vi "大富翁.vi"() -> ()   [LabVIEW 2014] (continued)
                                n1451 = property on="P2 棋子" class="Bool (strict)"("Left"=1540 ("Position:Left"), "Top"=112 ("Position:Top")) -> ()  [unwired: 2 in, 2 out]
                              }
                              frame 3 {
                                n1452 = local write "剩幾天 3"(2.0 ("剩幾天 3")) -> ()
                                n1453 = local write "位置 3"(13.0 ("位置 3")) -> ()
                                n1454 = property on="入獄 3" class="Bool (strict)"("Visible"=TRUE) -> ()  [unwired: 2 in, 2 out]
                                n1455 = property on="P3 棋子" class="Bool (strict)"("Left"=1503 ("Position:Left"), "Top"=144 ("Position:Top")) -> ()  [unwired: 2 in, 2 out]
                              }
                              frame 4 {
                                n1456 = local write "剩幾天 4"(2.0 ("剩幾天 4")) -> ()
                                n1457 = local write "位置 4"(13.0 ("位置 4")) -> ()
                                n1458 = property on="入獄 4" class="Bool (strict)"("Visible"=TRUE) -> ()  [unwired: 2 in, 2 out]
                                n1459 = property on="P4 棋子" class="Bool (strict)"("Left"=1540 ("Position:Left"), "Top"=144 ("Position:Top")) -> ()  [unwired: 2 in, 2 out]
                              }
                            }
                            n1460 = call "32入獄.vi"() -> ()  [unwired: 4 in]
                          }
                        }
                      }
                      frame True {
                        # "2~5"
                        n1461 = local read "換誰?"() -> (w868:dbl)
                        n1462 = case shown="1" w868 {
                          frame 0, Default {
                          }
                          frame 1 {
                            n1463 = local write "剩幾天 1"(3.0 ("剩幾天 1")) -> ()
                            n1464 = local write "位置 1"(13.0 ("位置 1")) -> ()
                            n1465 = property on="入獄 1" class="Bool (strict)"("Visible"=TRUE) -> ()  [unwired: 2 in, 2 out]
                            n1466 = property on="P1 棋子" class="Bool (strict)"("Left"=1503 ("Position:Left"), "Top"=112 ("Position:Top")) -> ()  [unwired: 2 in, 2 out]
                          }
                          frame 2 {
                            n1467 = local write "位置 2"(13.0 ("位置 2")) -> ()
                            n1468 = local write "剩幾天 2"(3.0 ("剩幾天 2")) -> ()
                            n1469 = property on="入獄 2" class="Bool (strict)"("Visible"=TRUE) -> ()  [unwired: 2 in, 2 out]
                            n1470 = property on="P2 棋子" class="Bool (strict)"("Left"=1540 ("Position:Left"), "Top"=112 ("Position:Top")) -> ()  [unwired: 2 in, 2 out]
                          }
                          frame 3 {
                            n1471 = local write "剩幾天 3"(3.0 ("剩幾天 3")) -> ()
                            n1472 = local write "位置 3"(13.0 ("位置 3")) -> ()
                            n1473 = property on="入獄 3" class="Bool (strict)"("Visible"=TRUE) -> ()  [unwired: 2 in, 2 out]
                            n1474 = property on="P3 棋子" class="Bool (strict)"("Left"=1503 ("Position:Left"), "Top"=144 ("Position:Top")) -> ()  [unwired: 2 in, 2 out]
                          }
                          frame 4 {
                            n1475 = local write "剩幾天 4"(3.0 ("剩幾天 4")) -> ()
                            n1476 = local write "位置 4"(13.0 ("位置 4")) -> ()
                            n1477 = property on="入獄 4" class="Bool (strict)"("Visible"=TRUE) -> ()  [unwired: 2 in, 2 out]
                            n1478 = property on="P4 棋子" class="Bool (strict)"("Left"=1540 ("Position:Left"), "Top"=144 ("Position:Top")) -> ()  [unwired: 2 in, 2 out]
                          }
                        }
                        n1479 = call "入獄3天.vi"() -> ()  [unwired: 4 in]
                      }
                    }
                  }
                  frame True {
                    # "0~2%"
                    n1480 = stacked-sequence {
                      tunnel: [_ w922] -> w889
                      frame #0 {
                        n1481 = local read "換誰?"() -> (w890:dbl)
                        n1482 = case shown="4" w890 {
                          frame 0, Default {
                          }
                          frame 1 {
                            n1483 = local write "剩幾天 1"(5.0 ("剩幾天 1")) -> ()
                            n1484 = local write "位置 1"(13.0 ("位置 1")) -> ()
                            n1485 = property on="入獄 1" class="Bool (strict)"("Visible"=TRUE) -> ()  [unwired: 2 in, 2 out]
                            n1486 = property on="P1 棋子" class="Bool (strict)"("Left"=1503 ("Position:Left"), "Top"=112 ("Position:Top")) -> ()  [unwired: 2 in, 2 out]
                          }
                          frame 2 {
                            n1487 = local write "位置 2"(13.0 ("位置 2")) -> ()
                            n1488 = local write "剩幾天 2"(5.0 ("剩幾天 2")) -> ()
                            n1489 = property on="入獄 2" class="Bool (strict)"("Visible"=TRUE) -> ()  [unwired: 2 in, 2 out]
                            n1490 = property on="P2 棋子" class="Bool (strict)"("Left"=1540 ("Position:Left"), "Top"=112 ("Position:Top")) -> ()  [unwired: 2 in, 2 out]
                          }
                          frame 3 {
                            n1491 = local write "剩幾天 3"(5.0 ("剩幾天 3")) -> ()
                            n1492 = local write "位置 3"(13.0 ("位置 3")) -> ()
                            n1493 = property on="入獄 3" class="Bool (strict)"("Visible"=TRUE) -> ()  [unwired: 2 in, 2 out]
                            n1494 = property on="P3 棋子" class="Bool (strict)"("Left"=1503 ("Position:Left"), "Top"=144 ("Position:Top")) -> ()  [unwired: 2 in, 2 out]
                          }
                          frame 4 {
                            n1495 = local write "剩幾天 4"(5.0 ("剩幾天 4")) -> ()
                            n1496 = local write "位置 4"(13.0 ("位置 4")) -> ()
                            n1497 = property on="入獄 4" class="Bool (strict)"("Visible"=TRUE) -> ()  [unwired: 2 in, 2 out]
                            n1498 = property on="P4 棋子" class="Bool (strict)"("Left"=1540 ("Position:Left"), "Top"=144 ("Position:Top")) -> ()  [unwired: 2 in, 2 out]
                          }
                        }
                        n1499 = case shown="1, Default" w890 {
                          tunnel: [w898 w899 w900 w901] -> w893
                          frame 1, Default {
                            n1500 = local read "玩家一財產"() -> (w898:dbl)
                          }
                          frame 2 {
                            n1501 = local read "玩家二財產"() -> (w899:dbl)
                          }
                          frame 3 {
                            n1502 = local read "玩家三財產"() -> (w900:dbl)
                          }
                          frame 4 {
                            n1503 = local read "玩家四財產"() -> (w901:dbl)
                          }
                        }
                        n1504 = Subtract(x=w893, y=2000.0) -> (x-y=w891:dbl)
                        n1505 = case shown="4" w890 {
                          tunnel: w891 -> [w894 w895 w896 w897]
                          frame 1, Default {
                            n1506 = local write "玩家一財產"(w894) -> ()
                          }
                          frame 2 {
                            n1507 = local write "玩家二財產"(w895) -> ()
                          }
                          frame 3 {
                            n1508 = local write "玩家三財產"(w896) -> ()
                          }
                          frame 4 {
                            n1509 = local write "玩家四財產"(w897) -> ()
                          }
                        }
                        n1510 = call "入獄5天.vi"() -> ()  [unwired: 4 in]
                      }
                      frame #1 {
                        n1511 = local read "換誰?"() -> (w924:dbl)
                        n1512 = case shown="1, Default" w924 {
                          tunnel: [w928 w929 w930 w931] -> w925
                          frame 1, Default {
                            n1513 = local read "玩家一財產"() -> (w928:dbl)
                          }
                          frame 2 {
                            n1514 = local read "玩家二財產"() -> (w929:dbl)
                          }
                          frame 3 {
                            n1515 = local read "玩家三財產"() -> (w930:dbl)
                          }
                          frame 4 {
                            n1516 = local read "玩家四財產"() -> (w931:dbl)
                          }
                        }
                        n1517 = Less Than 0?(x=w925) -> (x < 0?=w923:bool)
                        n1518 = case shown="True" w923 {
                          tunnel: [FALSE TRUE] -> w922
                          frame False {
                          }
                          frame True {
                            n1519 = call "破產了.vi"() -> ()  [unwired: 4 in]
                          }
                        }
                      }
                    }
                  }
                }
              }
              frame True {
                n1520 = local read "換誰?"() -> (w933:dbl)
                n1521 = case shown="4" w933 {
                  frame 0, Default {
                  }
                  frame 1 {
                    n1522 = local write "剩幾天 1"(2.0 ("剩幾天 1")) -> ()
                    n1523 = local write "位置 1"(13.0 ("位置 1")) -> ()
                    n1524 = property on="入獄 1" class="Bool (strict)"("Visible"=TRUE) -> ()  [unwired: 2 in, 2 out]
                    n1525 = property on="P1 棋子" class="Bool (strict)"("Left"=1503 ("Position:Left"), "Top"=112 ("Position:Top")) -> ()  [unwired: 2 in, 2 out]
                  }
                  frame 2 {
                    n1526 = local write "位置 2"(13.0 ("位置 2")) -> ()
                    n1527 = local write "剩幾天 2"(2.0 ("剩幾天 2")) -> ()
                    n1528 = property on="入獄 2" class="Bool (strict)"("Visible"=TRUE) -> ()  [unwired: 2 in, 2 out]
                    n1529 = property on="P2 棋子" class="Bool (strict)"("Left"=1540 ("Position:Left"), "Top"=112 ("Position:Top")) -> ()  [unwired: 2 in, 2 out]
                  }
                  frame 3 {
                    n1530 = local write "剩幾天 3"(2.0 ("剩幾天 3")) -> ()
                    n1531 = local write "位置 3"(13.0 ("位置 3")) -> ()
                    n1532 = property on="入獄 3" class="Bool (strict)"("Visible"=TRUE) -> ()  [unwired: 2 in, 2 out]
                    n1533 = property on="P3 棋子" class="Bool (strict)"("Left"=1503 ("Position:Left"), "Top"=144 ("Position:Top")) -> ()  [unwired: 2 in, 2 out]
                  }
                  frame 4 {
                    n1534 = local write "剩幾天 4"(2.0 ("剩幾天 4")) -> ()
                    n1535 = local write "位置 4"(13.0 ("位置 4")) -> ()
                    n1536 = property on="入獄 4" class="Bool (strict)"("Visible"=TRUE) -> ()  [unwired: 2 in, 2 out]
                    n1537 = property on="P4 棋子" class="Bool (strict)"("Left"=1540 ("Position:Left"), "Top"=144 ("Position:Top")) -> ()  [unwired: 2 in, 2 out]
                  }
                }
                n1538 = call "32入獄.vi"() -> ()  [unwired: 4 in]
              }
            }
          }
          frame 6 {
            n1539 = local read "宜蘭縣所有"() -> (w954:u32)
            n1540 = Equal?(x=w954, y=u32 16777215) -> (x = y?=w957:bool)
            n1541 = case shown="False" w957 {
              tunnel: w956 -> [w980 w1018]
              tunnel: [w970 FALSE] -> w955
              frame False {
                # "有主地"
                n1542 = local read "換誰?"() -> (w973:dbl)
                n1543 = local read "宜蘭縣所有"() -> (w960:u32)
                n1544 = call "數字轉顏色.vi"("數字"=w973) -> ("顏色數字"=w984:dbl)  [unwired: 2 in]
                n1545 = case shown="4" w973 {
                  tunnel: [w1013 w1014 w1015 w1016] -> w979
                  frame 1, Default {
                    n1546 = local read "玩家一財產"() -> (w1013:dbl)
                  }
                  frame 2 {
                    n1547 = local read "玩家二財產"() -> (w1014:dbl)
                  }
                  frame 3 {
                    n1548 = local read "玩家三財產"() -> (w1015:dbl)
                  }
                  frame 4 {
                    n1549 = local read "玩家四財產"() -> (w1016:dbl)
                  }
                }
                n1550 = Equal?(x=w960, y=w984) -> (x = y?=w983:bool)
                n1551 = local read "宜蘭縣所有"() -> (w961:u32)
                n1552 = local read "6旅4"() -> (w962:bool)
                n1553 = local read "6旅3"() -> (w963:bool)
                n1554 = local read "6旅2"() -> (w964:bool)
                n1555 = local read "6旅1"() -> (w965:bool)
                n1556 = local read "6房4"() -> (w966:bool)
                n1557 = local read "6房3"() -> (w967:bool)
                n1558 = local read "6房2"() -> (w968:bool)
                n1559 = local read "6房1"() -> (w969:bool)
                n1560 = call "房子數量.vi"("房子 1"=w969, "房子 2"=w968, "房子 3"=w967, "房子 4"=w966, "旅館 1"=w965, "旅館 2"=w964, "旅館 3"=w963, "旅館 4"=w962) -> ("房子數"=w982:dbl, "旅館數"=w981:dbl)  [unwired: 18 in]
                n1561 = call "顏色轉數字.vi"("顏色數字"=w961) -> ("數字"=w971:dbl)  [unwired: 2 in]
                n1562 = case shown="1, Default" w971 {
                  tunnel: [w989 w990 w991 w992] -> w975
                  frame 1, Default {
                    n1563 = local read "玩家一財產"() -> (w989:dbl)
                  }
                  frame 2 {
                    n1564 = local read "玩家二財產"() -> (w990:dbl)
                  }
                  frame 3 {
                    n1565 = local read "玩家三財產"() -> (w991:dbl)
                  }
                  frame 4 {
                    n1566 = local read "玩家四財產"() -> (w992:dbl)
                  }
                }
                n1567 = call "走到地.vi"("房子數量"=w982, "自己的地?"=w983, "旅館數量"=w981, "編號"=w980, "走到人財產"=w979) -> ("走到人-?"=w978:dbl, "蓋第幾棟"=w976:dbl, "地主+?"=w974:dbl, "破產?"=w970:bool)
                n1568 = Subtract(x=w979, y=w978) -> (x-y=w977:dbl)
                n1569 = Add(x=w974, y=w975) -> (x+y=w972:dbl)
                n1570 = case shown="1, Default" w971 {
                  tunnel: w972 -> [w985 w986 w987 w988]
                  frame 1, Default {
                    n1571 = local write "玩家一財產"(w985) -> ()
                  }
                  frame 2 {
                    n1572 = local write "玩家二財產"(w986) -> ()
                  }
                  frame 3 {
                    n1573 = local write "玩家三財產"(w987) -> ()
                  }
                  frame 4 {
                    n1574 = local write "玩家四財產"(w988) -> ()
                  }
                }
                n1575 = case shown="0, Default" w976 {
                  frame 0, Default {
                  }
                  frame 1 {
                    n1576 = flat-sequence {
                      frame #0 {
                        n1577 = local write "6房1"(TRUE ("1房1")) -> ()
                      }
                      frame #1 {
                        n1578 = property on="6房1" class="Bool (strict)"("Visible"=TRUE) -> ()  [unwired: 2 in, 2 out]
                      }
                    }
                  }
                  frame 2 {
                    n1579 = flat-sequence {
                      frame #0 {
                        n1580 = local write "6房2"(TRUE ("1房2")) -> ()
                      }
                      frame #1 {
                        n1581 = property on="6房2" class="Bool (strict)"("Visible"=TRUE ("1房2")) -> ()  [unwired: 2 in, 2 out]
                      }
                    }
                  }
                  frame 3 {
                    n1582 = flat-sequence {
                      frame #0 {
                        n1583 = local write "6房3"(TRUE) -> ()
                      }
                      frame #1 {
                        n1584 = property on="6房3" class="Bool (strict)"("Visible"=TRUE) -> ()  [unwired: 2 in, 2 out]
                      }
                    }
                  }
                  frame 4 {
                    n1585 = flat-sequence {
                      frame #0 {
                        n1586 = local write "6房4"(TRUE) -> ()
                      }
                      frame #1 {
                        n1587 = property on="6房4" class="Bool (strict)"("Visible"=TRUE) -> ()  [unwired: 2 in, 2 out]
                      }
                    }
                  }
                  frame 5 {
                    n1588 = flat-sequence {
                      frame #0 {
                        n1589 = local write "6旅1"(TRUE) -> ()
                      }
                      frame #1 {
                        n1590 = property on="6旅1" class="Bool (strict)"("Visible"=TRUE) -> ()  [unwired: 2 in, 2 out]
                      }
                    }
                  }
                  frame 6 {
                    n1591 = flat-sequence {
                      frame #0 {
                        n1592 = local write "6旅2"(TRUE) -> ()
                      }
                      frame #1 {
                        n1593 = property on="6旅2" class="Bool (strict)"("Visible"=TRUE) -> ()  [unwired: 2 in, 2 out]
                      }
                    }
                  }
                  frame 7 {
                    n1594 = flat-sequence {
                      frame #0 {
                        n1595 = local write "6旅3"(TRUE) -> ()
                      }
                      frame #1 {
                        n1596 = property on="6旅3" class="Bool (strict)"("Visible"=TRUE) -> ()  [unwired: 2 in, 2 out]
                      }
                    }
                  }
                  frame 8 {
                    n1597 = flat-sequence {
                      frame #0 {
                        n1598 = local write "6旅4"(TRUE) -> ()
                      }
                      frame #1 {
                        n1599 = property on="6旅4" class="Bool (strict)"("Visible"=TRUE) -> ()  [unwired: 2 in, 2 out]
                      }
                    }
                  }
                }
                n1600 = case shown="1, Default" w973 {
                  tunnel: w977 -> [w1009 w1010 w1011 w1012]
                  frame 1, Default {
                    n1601 = local write "玩家一財產"(w1009) -> ()
                  }
                  frame 2 {
                    n1602 = local write "玩家二財產"(w1010) -> ()
                  }
                  frame 3 {
                    n1603 = local write "玩家三財產"(w1011) -> ()
                  }
                  frame 4 {
                    n1604 = local write "玩家四財產"(w1012) -> ()
                  }
                }
              }
              frame True {
                # "無主地"
                n1605 = call "購買土地.vi"() -> ("確定 2"=w1019:bool)  [unwired: 3 in]
                n1606 = case shown="True" w1019 {
                  tunnel: w1018 -> [_ w1023]
                  frame False {
                    # "不買"
                  }
                  frame True {
                    # "要買"
                    n1607 = local read "換誰?"() -> (w1024:dbl)
                    n1608 = case shown="4" w1024 {
                      tunnel: [w1051 w1052 w1053 w1054] -> w1022
                      frame 1, Default {
                        n1609 = local read "玩家一財產"() -> (w1051:dbl)
                      }
                      frame 2 {
                        n1610 = local read "玩家二財產"() -> (w1052:dbl)
                      }
                      frame 3 {
                        n1611 = local read "玩家三財產"() -> (w1053:dbl)
                      }
                      frame 4 {
                        n1612 = local read "玩家四財產"() -> (w1054:dbl)
                      }
                    }
                    n1613 = call "各種價格.vi"("Numeric"=w1023) -> ("買空地"=w1021:dbl)  [unwired: 4 in, 5 out]
                    n1614 = Greater Or Equal?(x=w1022, y=w1021) -> (x >= y?=w1020:bool)
                    n1615 = case shown="True" w1020 {
                      tunnel: w1023 -> [_ w1025]
                      frame False {
                        # "錢不夠"
                        n1616 = call "錢不夠.vi"() -> ()  [unwired: 4 in]
                      }
                      frame True {
                        # "錢夠"
                        n1617 = local read "換誰?"() -> (w1026:dbl)
                        n1618 = case shown="4" w1026 {
                          selector: w1026 -> [w1030 w1036 w1042 w1048]
                          tunnel: w1025 -> [w1029 w1035 w1041 w1047]
                          frame 1, Default {
                            # "誰買了地"
                            n1619 = call "各種價格.vi"("Numeric"=w1029) -> ("買空地"=w1028:dbl)  [unwired: 4 in, 5 out]
                            n1620 = local read "玩家一財產"() -> (w1032:dbl)
                            n1621 = Subtract(x=w1032, y=w1028) -> (x-y=w1031:dbl)
                            n1622 = local write "玩家一財產"(w1031) -> ()
                            n1623 = call "數字轉顏色.vi"("數字"=w1030) -> ("顏色數字"=w1027:dbl)  [unwired: 2 in]
                            n1624 = local write "宜蘭縣所有"(w1027) -> ()
                            n1625 = local write "6宜蘭縣"(w1027) -> ()
                          }
                          frame 2 {
                            # "誰買了地"
                            n1626 = call "各種價格.vi"("Numeric"=w1035) -> ("買空地"=w1034:dbl)  [unwired: 4 in, 5 out]
                            n1627 = local read "玩家二財產"() -> (w1038:dbl)
                            n1628 = Subtract(x=w1038, y=w1034) -> (x-y=w1037:dbl)
                            n1629 = local write "玩家二財產"(w1037) -> ()
                            n1630 = call "數字轉顏色.vi"("數字"=w1036) -> ("顏色數字"=w1033:dbl)  [unwired: 2 in]
                            n1631 = local write "宜蘭縣所有"(w1033) -> ()
                            n1632 = local write "6宜蘭縣"(w1033) -> ()
                          }
                          frame 3 {
                            # "誰買了地"
                            n1633 = local read "玩家三財產"() -> (w1043:dbl)
                            n1634 = call "各種價格.vi"("Numeric"=w1041) -> ("買空地"=w1040:dbl)  [unwired: 4 in, 5 out]
                            n1635 = Subtract(x=w1043, y=w1040) -> (x-y=w1044:dbl)
                            n1636 = call "數字轉顏色.vi"("數字"=w1042) -> ("顏色數字"=w1039:dbl)  [unwired: 2 in]
                            n1637 = local write "玩家三財產"(w1044) -> ()
                            n1638 = local write "宜蘭縣所有"(w1039) -> ()
                            n1639 = local write "6宜蘭縣"(w1039) -> ()
                          }
                          frame 4 {
                            # "誰買了地"
                            n1640 = call "各種價格.vi"("Numeric"=w1047) -> ("買空地"=w1046:dbl)  [unwired: 4 in, 5 out]
                            n1641 = local read "玩家四財產"() -> (w1050:dbl)
                            n1642 = Subtract(x=w1050, y=w1046) -> (x-y=w1049:dbl)
                            n1643 = local write "玩家四財產"(w1049) -> ()
                            n1644 = call "數字轉顏色.vi"("數字"=w1048) -> ("顏色數字"=w1045:dbl)  [unwired: 2 in]
                            n1645 = local write "宜蘭縣所有"(w1045) -> ()
                            n1646 = local write "6宜蘭縣"(w1045) -> ()
                          }
                        }
                      }
                    }
                  }
                }
              }
            }
          }
          frame 7 {
            n1647 = local read "花蓮縣所有"() -> (w1055:u32)
            n1648 = Equal?(x=w1055, y=u32 16777215) -> (x = y?=w1058:bool)
            n1649 = case shown="False" w1058 {
              tunnel: w1057 -> [w1081 w1119]
              tunnel: [w1071 FALSE] -> w1056
              frame False {
                # "有主地"
                n1650 = local read "換誰?"() -> (w1074:dbl)
                n1651 = local read "花蓮縣所有"() -> (w1062:u32)
                n1652 = call "數字轉顏色.vi"("數字"=w1074) -> ("顏色數字"=w1085:dbl)  [unwired: 2 in]
                n1653 = case shown="4" w1074 {
                  tunnel: [w1114 w1115 w1116 w1117] -> w1080
                  frame 1, Default {
                    n1654 = local read "玩家一財產"() -> (w1114:dbl)
                  }
                  frame 2 {
                    n1655 = local read "玩家二財產"() -> (w1115:dbl)
                  }
                  frame 3 {
                    n1656 = local read "玩家三財產"() -> (w1116:dbl)
                  }
                  frame 4 {
                    n1657 = local read "玩家四財產"() -> (w1117:dbl)
                  }
                }
                n1658 = Equal?(x=w1062, y=w1085) -> (x = y?=w1084:bool)
                n1659 = local read "花蓮縣所有"() -> (w1061:u32)
                n1660 = local read "7旅4"() -> (w1070:bool)
                n1661 = local read "7旅3"() -> (w1069:bool)
                n1662 = local read "7旅2"() -> (w1068:bool)
                n1663 = local read "7旅1"() -> (w1067:bool)
                n1664 = local read "7房4"() -> (w1066:bool)
                n1665 = local read "7房3"() -> (w1065:bool)
                n1666 = local read "7房2"() -> (w1064:bool)
                n1667 = local read "7房1"() -> (w1063:bool)
                n1668 = call "房子數量.vi"("房子 1"=w1063, "房子 2"=w1064, "房子 3"=w1065, "房子 4"=w1066, "旅館 1"=w1067, "旅館 2"=w1068, "旅館 3"=w1069, "旅館 4"=w1070) -> ("房子數"=w1083:dbl, "旅館數"=w1082:dbl)  [unwired: 18 in]
                n1669 = call "顏色轉數字.vi"("顏色數字"=w1061) -> ("數字"=w1072:dbl)  [unwired: 2 in]
                n1670 = case shown="1, Default" w1072 {
                  tunnel: [w1090 w1091 w1092 w1093] -> w1076
                  frame 1, Default {
                    n1671 = local read "玩家一財產"() -> (w1090:dbl)
                  }
                  frame 2 {
                    n1672 = local read "玩家二財產"() -> (w1091:dbl)
                  }
                  frame 3 {
                    n1673 = local read "玩家三財產"() -> (w1092:dbl)
                  }
                  frame 4 {
                    n1674 = local read "玩家四財產"() -> (w1093:dbl)
                  }
                }
                n1675 = call "走到地.vi"("房子數量"=w1083, "自己的地?"=w1084, "旅館數量"=w1082, "編號"=w1081, "走到人財產"=w1080) -> ("走到人-?"=w1079:dbl, "蓋第幾棟"=w1077:dbl, "地主+?"=w1075:dbl, "破產?"=w1071:bool)
                n1676 = Subtract(x=w1080, y=w1079) -> (x-y=w1078:dbl)
                n1677 = Add(x=w1075, y=w1076) -> (x+y=w1073:dbl)
                n1678 = case shown="1, Default" w1072 {
                  tunnel: w1073 -> [w1086 w1087 w1088 w1089]
                  frame 1, Default {
                    n1679 = local write "玩家一財產"(w1086) -> ()
                  }
                  frame 2 {
                    n1680 = local write "玩家二財產"(w1087) -> ()
                  }
                  frame 3 {
                    n1681 = local write "玩家三財產"(w1088) -> ()
                  }
                  frame 4 {
                    n1682 = local write "玩家四財產"(w1089) -> ()
                  }
                }
                n1683 = case shown="6" w1077 {
                  frame 0, Default {
                  }
                  frame 1 {
                    n1684 = flat-sequence {
                      frame #0 {
                        n1685 = local write "7房1"(TRUE ("1房1")) -> ()
                      }
                      frame #1 {
                        n1686 = property on="7房1" class="Bool (strict)"("Visible"=TRUE) -> ()  [unwired: 2 in, 2 out]
                      }
                    }
                  }
                  frame 2 {
                    n1687 = flat-sequence {
                      frame #0 {
                        n1688 = local write "7房2"(TRUE ("1房2")) -> ()
                      }
                      frame #1 {
                        n1689 = property on="7房2" class="Bool (strict)"("Visible"=TRUE ("1房2")) -> ()  [unwired: 2 in, 2 out]
                      }
                    }
                  }
                  frame 3 {
                    n1690 = flat-sequence {
                      frame #0 {
                        n1691 = local write "7房3"(TRUE) -> ()
                      }
                      frame #1 {
                        n1692 = property on="7房3" class="Bool (strict)"("Visible"=TRUE) -> ()  [unwired: 2 in, 2 out]
                      }
                    }
                  }
                  frame 4 {
                    n1693 = flat-sequence {
                      frame #0 {
                        n1694 = local write "7房4"(TRUE) -> ()
                      }
                      frame #1 {
                        n1695 = property on="7房4" class="Bool (strict)"("Visible"=TRUE) -> ()  [unwired: 2 in, 2 out]
                      }
                    }
                  }
                  frame 5 {
                    n1696 = flat-sequence {
                      frame #0 {
                        n1697 = local write "7旅1"(TRUE) -> ()
                      }
                      frame #1 {
                        n1698 = property on="7旅1" class="Bool (strict)"("Visible"=TRUE) -> ()  [unwired: 2 in, 2 out]
                      }
                    }
                  }
                  frame 6 {
                    n1699 = flat-sequence {
                      frame #0 {
                        n1700 = local write "7旅2"(TRUE) -> ()
                      }
                      frame #1 {
                        n1701 = property on="7旅2" class="Bool (strict)"("Visible"=TRUE) -> ()  [unwired: 2 in, 2 out]
                      }
                    }
                  }
                  frame 7 {
                    n1702 = flat-sequence {
                      frame #0 {
                        n1703 = local write "7旅3"(TRUE) -> ()
                      }
                      frame #1 {
                        n1704 = property on="7旅3" class="Bool (strict)"("Visible"=TRUE) -> ()  [unwired: 2 in, 2 out]
                      }
                    }
                  }
                  frame 8 {
                    n1705 = flat-sequence {
                      frame #0 {
                        n1706 = local write "7旅4"(TRUE) -> ()
                      }
                      frame #1 {
                        n1707 = property on="7旅4" class="Bool (strict)"("Visible"=TRUE) -> ()  [unwired: 2 in, 2 out]
                      }
                    }
                  }
                }
                n1708 = case shown="1, Default" w1074 {
                  tunnel: w1078 -> [w1110 w1111 w1112 w1113]
                  frame 1, Default {
                    n1709 = local write "玩家一財產"(w1110) -> ()
                  }
                  frame 2 {
                    n1710 = local write "玩家二財產"(w1111) -> ()
                  }
                  frame 3 {
                    n1711 = local write "玩家三財產"(w1112) -> ()
                  }
                  frame 4 {
                    n1712 = local write "玩家四財產"(w1113) -> ()
                  }
                }
              }
              frame True {
                # "無主地"
                n1713 = call "購買土地.vi"() -> ("確定 2"=w1120:bool)  [unwired: 3 in]
                n1714 = case shown="True" w1120 {
                  tunnel: w1119 -> [_ w1124]
                  frame False {
                    # "不買"
                  }
                  frame True {
                    # "要買"
                    n1715 = local read "換誰?"() -> (w1125:dbl)
                    n1716 = case shown="4" w1125 {
                      tunnel: [w1152 w1153 w1154 w1155] -> w1123
                      frame 1, Default {
                        n1717 = local read "玩家一財產"() -> (w1152:dbl)
                      }
                      frame 2 {
                        n1718 = local read "玩家二財產"() -> (w1153:dbl)
                      }
                      frame 3 {
                        n1719 = local read "玩家三財產"() -> (w1154:dbl)
                      }
                      frame 4 {
                        n1720 = local read "玩家四財產"() -> (w1155:dbl)
                      }
                    }
                    n1721 = call "各種價格.vi"("Numeric"=w1124) -> ("買空地"=w1122:dbl)  [unwired: 4 in, 5 out]
                    n1722 = Greater Or Equal?(x=w1123, y=w1122) -> (x >= y?=w1121:bool)
                    n1723 = case shown="True" w1121 {
                      tunnel: w1124 -> [_ w1126]
                      frame False {
                        # "錢不夠"
                        n1724 = call "錢不夠.vi"() -> ()  [unwired: 4 in]
                      }
                      frame True {
                        # "錢夠"
                        n1725 = local read "換誰?"() -> (w1127:dbl)
                        n1726 = case shown="1, Default" w1127 {
                          selector: w1127 -> [w1131 w1137 w1143 w1149]
                          tunnel: w1126 -> [w1130 w1136 w1142 w1148]
                          frame 1, Default {
                            # "誰買了地"
                            n1727 = call "各種價格.vi"("Numeric"=w1130) -> ("買空地"=w1129:dbl)  [unwired: 4 in, 5 out]
                            n1728 = local read "玩家一財產"() -> (w1133:dbl)
                            n1729 = Subtract(x=w1133, y=w1129) -> (x-y=w1132:dbl)
                            n1730 = local write "玩家一財產"(w1132) -> ()
                            n1731 = call "數字轉顏色.vi"("數字"=w1131) -> ("顏色數字"=w1128:dbl)  [unwired: 2 in]
                            n1732 = local write "7花蓮縣"(w1128) -> ()
                            n1733 = local write "花蓮縣所有"(w1128) -> ()
                          }
                          frame 2 {
                            # "誰買了地"
                            n1734 = call "各種價格.vi"("Numeric"=w1136) -> ("買空地"=w1135:dbl)  [unwired: 4 in, 5 out]
                            n1735 = local read "玩家二財產"() -> (w1139:dbl)
                            n1736 = Subtract(x=w1139, y=w1135) -> (x-y=w1138:dbl)
                            n1737 = local write "玩家二財產"(w1138) -> ()
                            n1738 = call "數字轉顏色.vi"("數字"=w1137) -> ("顏色數字"=w1134:dbl)  [unwired: 2 in]
                            n1739 = local write "7花蓮縣"(w1134) -> ()
                            n1740 = local write "花蓮縣所有"(w1134) -> ()
                          }
                          frame 3 {
                            # "誰買了地"
                            n1741 = local read "玩家三財產"() -> (w1144:dbl)
                            n1742 = call "各種價格.vi"("Numeric"=w1142) -> ("買空地"=w1141:dbl)  [unwired: 4 in, 5 out]
                            n1743 = Subtract(x=w1144, y=w1141) -> (x-y=w1145:dbl)
                            n1744 = call "數字轉顏色.vi"("數字"=w1143) -> ("顏色數字"=w1140:dbl)  [unwired: 2 in]
                            n1745 = local write "玩家三財產"(w1145) -> ()
                            n1746 = local write "7花蓮縣"(w1140) -> ()
                            n1747 = local write "花蓮縣所有"(w1140) -> ()
                          }
                          frame 4 {
                            # "誰買了地"
                            n1748 = call "各種價格.vi"("Numeric"=w1148) -> ("買空地"=w1147:dbl)  [unwired: 4 in, 5 out]
                            n1749 = local read "玩家四財產"() -> (w1151:dbl)
                            n1750 = Subtract(x=w1151, y=w1147) -> (x-y=w1150:dbl)
                            n1751 = local write "玩家四財產"(w1150) -> ()
                            n1752 = call "數字轉顏色.vi"("數字"=w1149) -> ("顏色數字"=w1146:dbl)  [unwired: 2 in]
                            n1753 = local write "7花蓮縣"(w1146) -> ()
                            n1754 = local write "花蓮縣所有"(w1146) -> ()
                          }
                        }
                      }
                    }
                  }
                }
              }
            }
          }
          frame 8, 24, 35 {
            # "機會"
            n1755 = local read "白色恐怖?"() -> (w1157:bool)
            n1756 = case shown="False" w1157 {
              tunnel: [w1159 FALSE] -> w1156
              frame False {
                # "非白色恐怖"
                n1757 = Random Number (0-1)() -> (number: 0 to 1=w1164:dbl)
                n1758 = Multiply(x=w1164, y=100.0) -> (x*y=w1160:dbl)
                n1759 = Less?(x=w1160, y=1.0) -> (x < y?=w1161:bool)
                n1760 = case shown="False" w1161 {
                  tunnel: w1160 -> [w1166 _]
                  tunnel: [w1165 w1435] -> w1159
                  frame False {
                    # "2~100"
                    n1761 = Less?(x=w1166, y=3.0) -> (x < y?=w1167:bool)
                    n1762 = case shown="False" w1167 {
                      tunnel: w1166 -> [w1170 _]
                      tunnel: [w1169 FALSE] -> w1165
                      frame False {
                        # "5~100"
                        n1763 = Less?(x=w1170, y=6.0) -> (x < y?=w1171:bool)
                        n1764 = case shown="False" w1171 {
                          tunnel: w1170 -> [w1174 _]
                          tunnel: [w1173 FALSE] -> w1169
                          frame False {
                            # "10~100"
                            n1765 = Less?(x=w1174, y=30.0) -> (x < y?=w1175:bool)
                            n1766 = case shown="False" w1175 {
                              tunnel: w1174 -> [w1178 _]
                              tunnel: [w1177 FALSE] -> w1173
                              frame False {
                                # "30~100"
                                n1767 = Less?(x=w1178, y=45.0) -> (x < y?=w1179:bool)
                                n1768 = case shown="False" w1179 {
                                tunnel: w1178 -> [w1182 _]
                                tunnel: [w1181 FALSE] -> w1177
                                frame False {
                                # "45~100"
                                n1769 = Less?(x=w1182, y=54.0) -> (x < y?=w1183:bool)
                                n1770 = case shown="False" w1183 {
                                tunnel: w1182 -> [w1186 _]
                                tunnel: [w1185 FALSE] -> w1181
                                frame False {
                                # "54~100"
                                n1771 = Less?(x=w1186, y=58.0) -> (x < y?=w1187:bool)
                                n1772 = case shown="False" w1187 {
                                tunnel: w1186 -> [w1190 _]
                                tunnel: [w1189 FALSE] -> w1185
                                frame False {
                                # "58~100"
                                n1773 = Less?(x=w1190, y=60.0) -> (x < y?=w1191:bool)
                                n1774 = case shown="False" w1191 {
                                tunnel: w1190 -> [w1194 _]
                                tunnel: [w1193 FALSE] -> w1189
                                frame False {
                                # "58~60"
                                n1775 = Less?(x=w1194, y=74.0) -> (x < y?=w1195:bool)
                                n1776 = case shown="False" w1195 {
                                tunnel: w1194 -> [w1198 _]
                                tunnel: [w1197 w1303] -> w1193
                                frame False {
                                # "60~84"
                                n1777 = Less?(x=w1198, y=84.0) -> (x < y?=w1199:bool)
                                n1778 = case shown="False" w1199 {
                                tunnel: w1198 -> [w1202 _]
                                tunnel: [w1201 w1280] -> w1197
                                frame False {
                                # "84~94"
                                n1779 = Less?(x=w1202, y=94.0) -> (x < y?=w1203:bool)
                                n1780 = case shown="False" w1203 {
                                tunnel: w1202 -> [w1206 _]
                                tunnel: [w1205 w1257] -> w1201
                                frame False {
                                # "94~99"
                                n1781 = Less?(x=w1206, y=99.0) -> (x < y?=w1207:bool)
                                n1782 = case shown="True" w1207 {
                                tunnel: w1206 -> [_ _]
                                tunnel: [w1209 w1234] -> w1205
                                frame False {
                                n1783 = stacked-sequence {
                                tunnel: [_ w1231] -> w1209
                                frame #0 {
                                n1784 = local read "玩家三財產"() -> (w1213:dbl)
                                n1785 = local read "玩家四財產"() -> (w1211:dbl)
                                n1786 = local read "玩家一財產"() -> (w1217:dbl)
                                n1787 = local read "玩家二財產"() -> (w1215:dbl)
                                n1788 = Subtract(x=w1211, y=3000.0) -> (x-y=w1210:dbl)
                                n1789 = Subtract(x=w1217, y=3000.0) -> (x-y=w1216:dbl)
                                n1790 = Subtract(x=w1215, y=3000.0) -> (x-y=w1214:dbl)
                                n1791 = Subtract(x=w1213, y=3000.0) -> (x-y=w1212:dbl)
                                n1792 = local write "玩家一財產"(w1216) -> ()
                                n1793 = local write "玩家二財產"(w1214) -> ()
                                n1794 = local write "玩家四財產"(w1210) -> ()
                                n1795 = local write "玩家三財產"(w1212) -> ()
                                n1796 = call "機會全部-3000.vi"() -> ()  [unwired: 4 in]
                                }
                                frame #1 {
                                n1797 = local read "玩家四財產"() -> (w1230:dbl)
                                n1798 = local read "玩家三財產"() -> (w1229:dbl)
                                n1799 = local read "玩家二財產"() -> (w1228:dbl)
                                n1800 = local read "玩家一財產"() -> (w1227:dbl)
                                n1801 = Less Than 0?(x=w1230) -> (x < 0?=w1226:bool)
                                n1802 = Less Than 0?(x=w1228) -> (x < 0?=w1224:bool)
                                n1803 = Less Than 0?(x=w1229) -> (x < 0?=w1225:bool)
                                n1804 = Less Than 0?(x=w1227) -> (x < 0?=w1223:bool)
                                n1805 = Compound Arithmetic op=OR(w1226, w1225, w1224, w1223) -> (w1222:bool)
                                n1806 = case shown="True" w1222 {
                                tunnel: [FALSE TRUE] -> w1231
                                frame False {
                                }
                                frame True {
                                n1807 = call "破產了.vi"() -> ()  [unwired: 4 in]
                                }
                                }
                                }
                                }
                                }
                                frame True {
                                n1808 = stacked-sequence {
                                tunnel: [_ w1247] -> w1234
                                frame #0 {
                                n1809 = call "機會-3000.vi"() -> ()  [unwired: 4 in]
                                n1810 = local read "換誰?"() -> (w1235:dbl)
                                n1811 = case shown="1, Default" w1235 {
                                tunnel: [w1243 w1244 w1245 w1246] -> w1236
                                frame 1, Default {
                                n1812 = local read "玩家一財產"() -> (w1243:dbl)
                                }
                                frame 2 {
                                n1813 = local read "玩家二財產"() -> (w1244:dbl)
                                }
                                frame 3 {
                                n1814 = local read "玩家三財產"() -> (w1245:dbl)
                                }
                                frame 4 {
                                n1815 = local read "玩家四財產"() -> (w1246:dbl)
                                }
                                }
                                n1816 = Subtract(x=w1236, y=3000.0) -> (x-y=w1238:dbl)
                                n1817 = case shown="1, Default" w1235 {
                                tunnel: w1238 -> [w1239 w1240 w1241 w1242]
                                frame 1, Default {
                                n1818 = local write "玩家一財產"(w1239) -> ()
                                }
                                frame 2 {
                                n1819 = local write "玩家二財產"(w1240) -> ()
                                }
                                frame 3 {
                                n1820 = local write "玩家三財產"(w1241) -> ()
                                }
                                frame 4 {
                                n1821 = local write "玩家四財產"(w1242) -> ()
                                }
                                }
                                }
                                frame #1 {
                                n1822 = local read "換誰?"() -> (w1249:dbl)
                                n1823 = case shown="1, Default" w1249 {
                                tunnel: [w1253 w1254 w1255 w1256] -> w1250
                                frame 1, Default {
                                n1824 = local read "玩家一財產"() -> (w1253:dbl)
                                }
                                frame 2 {
                                n1825 = local read "玩家二財產"() -> (w1254:dbl)
                                }
                                frame 3 {
                                n1826 = local read "玩家三財產"() -> (w1255:dbl)
                                }
                                frame 4 {
                                n1827 = local read "玩家四財產"() -> (w1256:dbl)
                                }
                                }
                                n1828 = Less Than 0?(x=w1250) -> (x < 0?=w1248:bool)
                                n1829 = case shown="True" w1248 {
                                tunnel: [FALSE TRUE] -> w1247
                                frame False {
                                }
                                frame True {
                                n1830 = call "破產了.vi"() -> ()  [unwired: 4 in]
                                }
                                }
                                }
                                }
                                }
                                }
                                }
                                frame True {
                                n1831 = stacked-sequence {
                                tunnel: [_ w1270] -> w1257
                                frame #0 {
                                n1832 = call "機會-2000.vi"() -> ()  [unwired: 4 in]
                                n1833 = local read "換誰?"() -> (w1258:dbl)
                                n1834 = case shown="1, Default" w1258 {
                                tunnel: [w1266 w1267 w1268 w1269] -> w1259
                                frame 1, Default {
                                n1835 = local read "玩家一財產"() -> (w1266:dbl)
                                }
                                frame 2 {
                                n1836 = local read "玩家二財產"() -> (w1267:dbl)
                                }
                                frame 3 {
                                n1837 = local read "玩家三財產"() -> (w1268:dbl)
                                }
                                frame 4 {
                                n1838 = local read "玩家四財產"() -> (w1269:dbl)
                                }
                                }
                                n1839 = Subtract(x=w1259, y=2000.0) -> (x-y=w1261:dbl)
                                n1840 = case shown="1, Default" w1258 {
                                tunnel: w1261 -> [w1262 w1263 w1264 w1265]
                                frame 1, Default {
                                n1841 = local write "玩家一財產"(w1262) -> ()
                                }
                                frame 2 {
                                n1842 = local write "玩家二財產"(w1263) -> ()
                                }
                                frame 3 {
                                n1843 = local write "玩家三財產"(w1264) -> ()
                                }
                                frame 4 {
                                n1844 = local write "玩家四財產"(w1265) -> ()
                                }
                                }
                                }
                                frame #1 {
                                n1845 = local read "換誰?"() -> (w1272:dbl)
                                n1846 = case shown="1, Default" w1272 {
                                tunnel: [w1276 w1277 w1278 w1279] -> w1273
                                frame 1, Default {
                                n1847 = local read "玩家一財產"() -> (w1276:dbl)
                                }
                                frame 2 {
                                n1848 = local read "玩家二財產"() -> (w1277:dbl)
                                }
                                frame 3 {
                                n1849 = local read "玩家三財產"() -> (w1278:dbl)
                                }
                                frame 4 {
                                n1850 = local read "玩家四財產"() -> (w1279:dbl)
                                }
                                }
                                n1851 = Less Than 0?(x=w1273) -> (x < 0?=w1271:bool)
                                n1852 = case shown="True" w1271 {
                                tunnel: [FALSE TRUE] -> w1270
                                frame False {
                                }
                                frame True {
                                n1853 = call "破產了.vi"() -> ()  [unwired: 4 in]
                                }
                                }
                                }
                                }
                                }
                                }
                                }
                                frame True {
                                n1854 = stacked-sequence {
                                tunnel: [_ w1293] -> w1280
                                frame #0 {
                                n1855 = call "機會-1000.vi"() -> ()  [unwired: 4 in]
                                n1856 = local read "換誰?"() -> (w1281:dbl)
                                n1857 = case shown="1, Default" w1281 {
                                tunnel: [w1289 w1290 w1291 w1292] -> w1282
                                frame 1, Default {
                                n1858 = local read "玩家一財產"() -> (w1289:dbl)
                                }
                                frame 2 {
                                n1859 = local read "玩家二財產"() -> (w1290:dbl)
                                }
                                frame 3 {
                                n1860 = local read "玩家三財產"() -> (w1291:dbl)
                                }
                                frame 4 {
                                n1861 = local read "玩家四財產"() -> (w1292:dbl)
                                }
                                }
                                n1862 = Subtract(x=w1282, y=1000.0) -> (x-y=w1284:dbl)
                                n1863 = case shown="1, Default" w1281 {
                                tunnel: w1284 -> [w1285 w1286 w1287 w1288]
                                frame 1, Default {
                                n1864 = local write "玩家一財產"(w1285) -> ()
                                }
                                frame 2 {
                                n1865 = local write "玩家二財產"(w1286) -> ()
                                }
                                frame 3 {
                                n1866 = local write "玩家三財產"(w1287) -> ()
                                }
                                frame 4 {
                                n1867 = local write "玩家四財產"(w1288) -> ()
                                }
                                }
                                }
                                frame #1 {
                                n1868 = local read "換誰?"() -> (w1295:dbl)
                                n1869 = case shown="1, Default" w1295 {
                                tunnel: [w1299 w1300 w1301 w1302] -> w1296
                                frame 1, Default {
                                n1870 = local read "玩家一財產"() -> (w1299:dbl)
                                }
                                frame 2 {
                                n1871 = local read "玩家二財產"() -> (w1300:dbl)
                                }
                                frame 3 {
                                n1872 = local read "玩家三財產"() -> (w1301:dbl)
                                }
                                frame 4 {
                                n1873 = local read "玩家四財產"() -> (w1302:dbl)
                                }
                                }
                                n1874 = Less Than 0?(x=w1296) -> (x < 0?=w1294:bool)
                                n1875 = case shown="True" w1294 {
                                tunnel: [FALSE TRUE] -> w1293
                                frame False {
                                }
                                frame True {
                                n1876 = call "破產了.vi"() -> ()  [unwired: 4 in]
                                }
                                }
                                }
                                }
                                }
                                }
                                }
                                frame True {
